vi "PSDATA_Variant To DBL.vi"(9 "error in":errorcluster, 10 "Value":variant) -> (1 "error out":errorcluster, 2 "Value":string, 4 "DBL":dbl)   [LabVIEW 2016]
doc: "Developer：YDX"
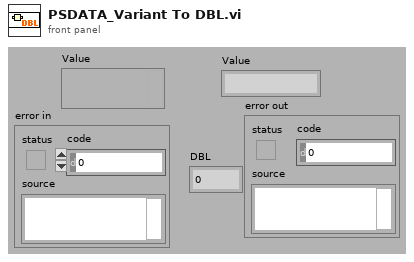
[diagram p1: front panel]
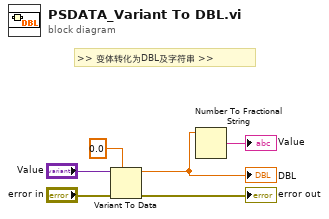
[diagram p0: block diagram]
diagram:
  # ">> 变体转化为DBL及字符串 >>"
  n1 = Variant To Data(error in="error in", type=0.0 ("Str"), Variant="Value") -> (data=w1:dbl, error out=→"error out":errorcluster)
  "DBL" <- w1
  n2 = Number To Fractional String(number=w1) -> (F-format string=→"Value":string)  [unwired: 3 in]
